vi "Initialize.vi"(8 "error in (no error)":errorcluster, 11 "INI in":refnum<class "Projects-INI.lvclass">) -> (0 "error out":errorcluster, 3 "INI out":refnum<class "Projects-INI.lvclass">)   [LabVIEW 2020, in "Projects-INI.lvclass"]
doc: "Perform any initialization actions necessary for the specific implementations of the class.\nThis implementation clears the Map by writing an empty Map to the project data.\n\n03/2025 Erich Schlieper"
uses:
  Projects-INI.lvclass
  <vilib>/Utility/sysdir.llb/System Directory Type.ctl
  Projects-INI.lvclass/Projects-INI.ctl
  Parent/Projects.lvclass
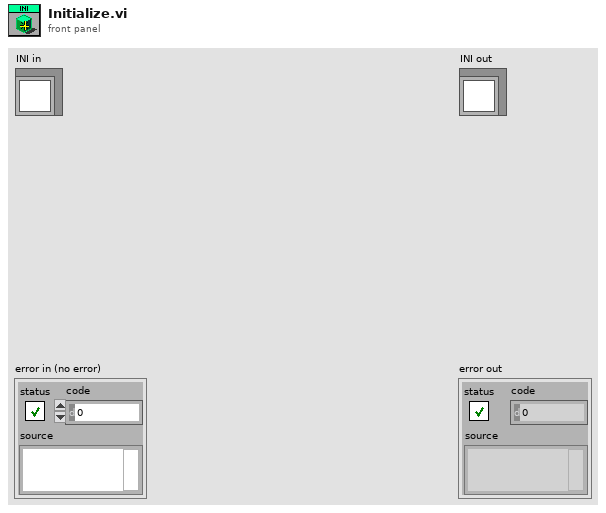
[diagram p1: front panel]
types:
  T1 = typedef "System Directory Type.ctl" = i32
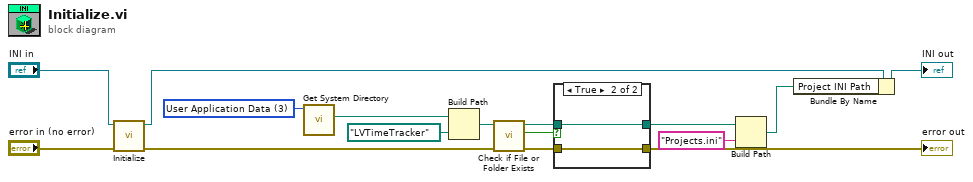
[diagram p0: block diagram]
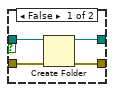
[diagram p2: hidden frame]
diagram:
  w13 = T1 3 items=["User Home"=0, "User Desktop"=1, "User Documents"=2, "User Application Data"=3, "User Preferences"=4, "User Temporary"=5, "Public Documents"=6, "Public Application Data"=7, "Public Preferences"=8, "Public Cache"=13, "System Core Libraries"=9, "System Installed Libraries"=10, "Application Files"=11, "Boot Volume Root"=12] ("system directory type")
  n1 = call-parent "Initialize.vi"("error in (no error)"="error in (no error)", "Projects in"="INI in") -> ("error out"=w3:errorcluster, "Projects out"=w16:refnum<class "Projects-INI.lvclass">)  [unwired: 8 in]
  n2 = call <vilib>:"Get System Directory.vi"("system directory type"=w13) -> ("system directory"=w12:path)  [unwired: 10 in]
  n3 = Build Path(base path=w12, name or relative path=path "LVTimeTracker") -> (appended path=w10:path)
  n4 = call <vilib>:"Check if File or Folder Exists.vi"("error in (no error)"=w3, "path"=w10) -> ("error out"=w7:errorcluster, "file or folder exists?"=w9:bool, "dup path"=w8:path)  [unwired: 7 in]
  n5 = case shown="True" w9 {
    tunnel: w8 -> [w20 w22]
    tunnel: w7 -> [w19 w21]
    tunnel: [w18 w21] -> w1
    tunnel: [w17 w22] -> w6
    frame False {
      n6 = Create Folder(path (use dialog)=w20, error in=w19) -> (created path=w17:path, error out=w18:errorcluster)  [unwired: 1 in, 1 out]
    }
    frame True {
    }
  }
  "error out" <- w1
  n7 = Build Path(base path=w6, name or relative path="Projects.ini") -> (appended path=w2:path)
  n8 = Bundle By Name(cluster=w16, "Project INI Path"=w2) -> (→"INI out":refnum<class "Projects-INI.lvclass">)
